vi "12-alt.vi"() -> ()   [LabVIEW 2021]
panel:
  in  "#divisors":i32
  out "Numeric":i32
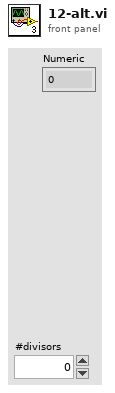
[diagram p1: front panel]
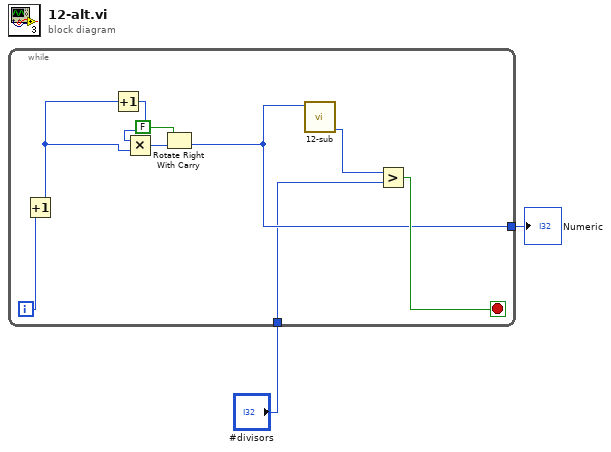
[diagram p0: block diagram]
diagram:
  n1 = while {
    tunnel: [w4] -> w2
    tunnel: "#divisors" -> [w3]
    i -> [w11]
    stop <- w9 stop-if-true
    n2 = Increment(x=w11) -> (x+1=w7:i32)
    n3 = Increment(x=w7) -> (x+1=w8:i32)
    n4 = Multiply(x=w8, y=w7) -> (x*y=w6:i32)
    n5 = Rotate Right With Carry(2:w6, 3:FALSE ("carry")) -> (0:w4:i32)  [unwired: 1 out]
    n6 = call "12-sub.vi"("Number"=w4) -> ("number of divisors"=w10:i32)  [unwired: 9 in, 1 out]
    n7 = Greater?(x=w10, y=w3) -> (0:w9:bool)
  }
  "Numeric" <- w2
